vi "ConnectToPLC.vi"(9 "sDataDir":string, 10 "ipAddr":string) -> (0 "error out":errorcluster, 1 "ExitCode":i32(ring) items=["Ok"=0, "ErrorCreateApplication"=17, "ErrorDiscoverEndpoints"=18, "ErrorCreateSession"=19, "ErrorBrowseNamespace"=20, "ErrorCreateSubscription"=21, "ErrorMonitoredItem"=22, "ErrorAddSubscription"=23, "ErrorRunning"=24, "ErrorNoKeepAlive"=48, "ErrorNoSecurityFile"=49, "ErrorInvalidCommandLine"=256], 2 "Handle":refnum<k24>)   [LabVIEW 2019]
uses:
  F:/src/HUTCDLSVN/Machine/CDL0100/TagEngine/LVOPCUA.NET/LVOPC.NETInterface/bin/Release/LVOPC.NETInterface.dll
  LVOPCUA.NET/LVOPC.NETInterface/bin/Release/LVOPC.NETInterface.dll
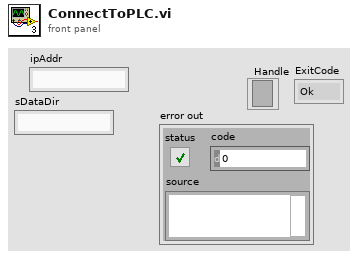
[diagram p1: front panel]
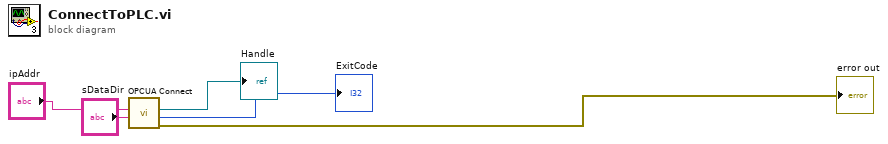
[diagram p0: block diagram]
diagram:
  n1 = call "OPCUA Connect.vi"("sDataDir"="sDataDir", "ipAddr"="ipAddr") -> ("error out"=→"error out":errorcluster, "ExitCode"=→"ExitCode":i32, "Handle"=→"Handle":refnum<k24>)  [unwired: 7 in]
